vi "ti2_getZEsc.vi"(8 "error in (no error)":errorcluster) -> (0 "error out":errorcluster, 3 "Escape Z?":bool)   [LabVIEW 2023, in "ti2lv.lvlib"]
uses:
  ti2lv.lvlib
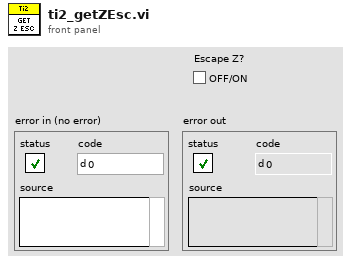
[diagram p1: front panel]
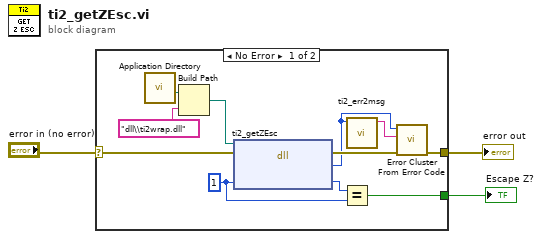
[diagram p0: block diagram]
diagram:
  n1 = case shown="No Error" "error in (no error)" {
    selector: "error in (no error)" -> [w13 w15]
    tunnel: [w14 w15] -> w2
    tunnel: [w4 _] -> w1
    frame No Error {
      w5 = 1 ("filterPos")
      n2 = call <vilib>:"Application Directory.vi"() -> ("Application Directory"=w8:path)
      n3 = Build Path(base path=w8, name or relative path="dll\\ti2wrap.dll") -> (appended path=w7:path)
      n4 = dll-call lib="C:/FlashGordon/Development/dll/ti2wrap.dll" fn="ti2_getZEsc"(path in=w7, error in=w13, "setting"=w5) -> (error out=w12:errorcluster, "return type"=w11:i32, "setting"=w6:i32)  [unwired: 1 in, 1 out]
      n5 = Equal?(x=w6, y=w5) -> (x = y?=w4:bool)
      n6 = call "ti2_err2msg.vi"("Error Code"=w11) -> ("Error Message"=w10:string)  [unwired: 10 in]
      n7 = call <vilib>:"Error Cluster From Error Code.vi"("error in (no error)"=w12, "error message (\"\")"=w10, "error code (0)"=w11) -> ("error out"=w14:errorcluster)  [unwired: 6 in]
    }
    frame Error {
    }
  }
  "error out" <- w2
  "Escape Z?" <- w1
